vi "Read 2019 SweepControl JSON.vi"(8 "error in (no error)":errorcluster, 11 "json file":path) -> (0 "error out":errorcluster, 3 "data":T1)   [LabVIEW 2016]
uses:
  <vilib>/addons/_JKI.lib/Serialization/JSON/JKI JSON Serialization.lvlib
panel:
  out "text":string
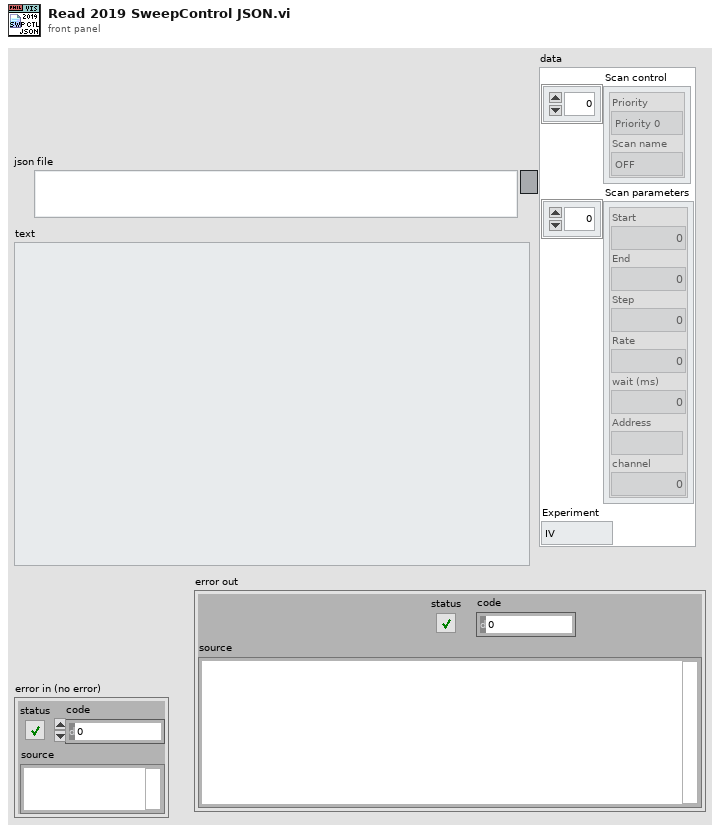
[diagram p1: front panel]
types:
  T1 = cluster{"Scan control":cluster{"Priority":enum16{"Priority 0", "Priority 1", "Priority 2", "Priority 3", "Priority 4", "Priority 5"}, "Scan name":enum16{"OFF", "DSA_Vsg2", "DSA_Vsg3", "DSA_Vbg", "DSA_Vsg1", "DSA_freq", "DSA_Vamp", "time", "Lockin Amplitude", "Lockin Frequency", "Lockin Bias", "Delay", "Strain", "DAQ Bias", "Magnet Field", "Temperature", "MW f1", "MW f2", "MW Amplitude1", "MW Amplitude2"}}[], "Scan parameters":cluster{"Start":dbl, "End":dbl, "Step":dbl, "Rate":dbl, "wait (ms)":u32, "Address":string, "channel":i32}[], "Experiment":enum16{"IV", "IV_Fast", "IV_Sweep", "THz_DelayLine", "Lockin_Vsg", "Lockin_Sweep", "Lockin_Time", "AI WFM time", "Lockin (experimental)"}}
  T2 = cluster{"Scan control":cluster{"Priority":enum16{"Priority 0", "Priority 1", "Priority 2", "Priority 3", "Priority 4", "Priority 5"}, "Scan name":enum16{"OFF", "DSA_Vsg2", "DSA_Vbg", "DSA_Vsg1", "DSA_freq", "DSA_Vamp", "time", "Lockin Amplitude", "Lockin Frequency", "Lockin Bias", "Delay", "Strain", "DAQ Bias", "Magnet Field", "Temperature", "MW f1", "MW f2", "MW Amplitude1", "MW Amplitude2"}}[], "Scan parameters":cluster{"Start":dbl, "End":dbl, "Step":dbl, "Rate":dbl, "wait (ms)":u32, "Address":string, "channel":i32}[], "Experiment":enum16{"IV", "IV_Fast", "IV_Sweep", "THz_DelayLine", "Lockin_Vsg", "Lockin_Sweep", "Lockin_Time", "AI WFM time", "Lockin (experimental)"}}
  T3 = cluster{"Experiment":enum16{"IV", "IV_Fast", "IV_Sweep", "THz_DelayLine", "Lockin_Vsg", "Lockin_Sweep", "Lockin_Time", "AI WFM time", "Lockin (experimental)"}, "Repeat Experiment":i32, "Scan control":cluster{"Priority":enum16{"Priority 0", "Priority 1", "Priority 2", "Priority 3", "Priority 4", "Priority 5"}, "Scan name":enum16{"OFF", "time", "Lockin Amplitude", "Lockin Frequency", "Lockin Bias", "Delay", "Strain", "DAQ Bias", "Magnet Field", "Temperature", "MW f1", "MW f2", "MW Amplitude1", "MW Amplitude2"}}[], "Scan parameters":cluster{"Start":dbl, "End":dbl, "Step":dbl, "Rate":dbl, "wait (ms/mK)":u32, "Address":string, "channel":i32}[]}
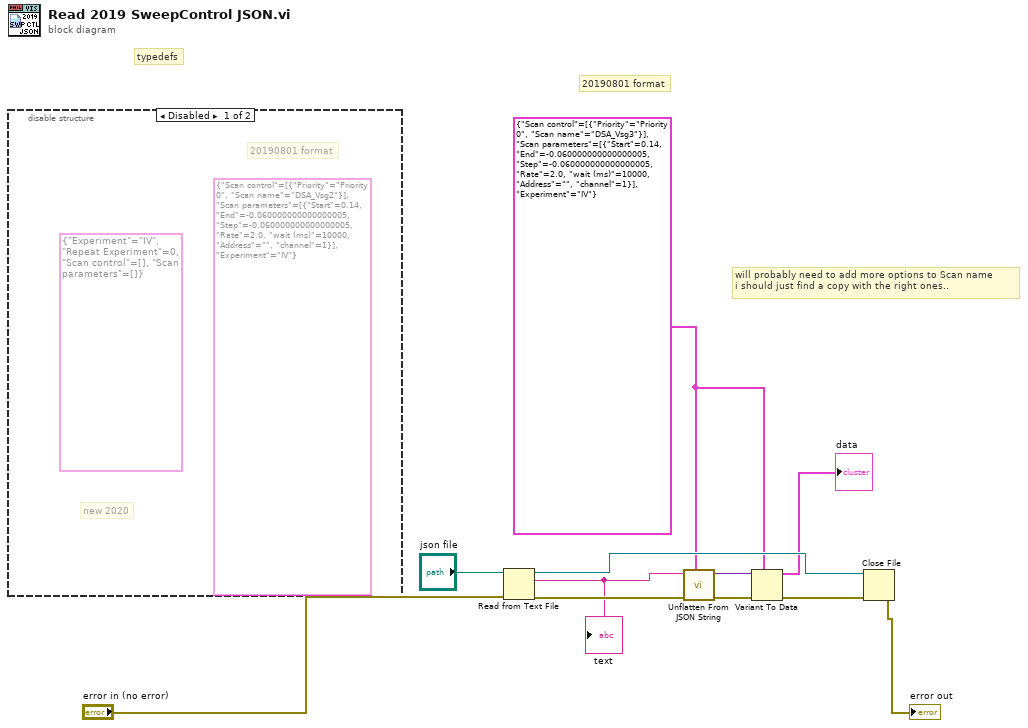
[diagram p0: block diagram]
diagram:
  w4 = T1 {"Scan control"=[{"Priority"=enum."Priority 0", "Scan name"=enum."DSA_Vsg3"}], "Scan parameters"=[{"Start"=0.14, "End"=-0.060000000000000005, "Step"=-0.060000000000000005, "Rate"=2.0, "wait (ms)"=10000, "Address"="", "channel"=1}], "Experiment"=enum."IV"} ("data")
  # "will probably need to add more options to Scan name\ni should just find a copy with the right ones.."
  # "20190801 format"
  # "typedefs"
  n1 = disable-structure shown="Disabled" {
    frame Disabled {
      (unwired) T2 {"Scan control"=[{"Priority"=enum."Priority 0", "Scan name"=enum."DSA_Vsg2"}], "Scan parameters"=[{"Start"=0.14, "End"=-0.060000000000000005, "Step"=-0.060000000000000005, "Rate"=2.0, "wait (ms)"=10000, "Address"="", "channel"=1}], "Experiment"=enum."IV"} ("data")
      (unwired) T3 {"Experiment"=enum."IV", "Repeat Experiment"=0, "Scan control"=[], "Scan parameters"=[]} ("data")
      # "20190801 format"
      # "new 2020"
    }
    frame Enabled {
    }
  }
  n2 = Read from Text File(file (use dialog)="json file", error in="error in (no error)") -> (refnum out=w7:refnum<file>, text=w6:string, error out=w11:errorcluster)  [unwired: 2 in, 1 out]
  "text" <- w6
  n3 = call <vilib>:"Unflatten From JSON String.vi"("Type and Defaults"=w4, "error in (no error)"=w11, "JSON String"=w6) -> ("error out"=w3:errorcluster, "Variant"=w5:variant)  [unwired: 7 in]
  n4 = Variant To Data(error in=w3, type=w4, Variant=w5) -> (data=→"data":T1, error out=w2:errorcluster)
  n5 = Close File(refnum=w7, error in=w2) -> (error out=→"error out":errorcluster)  [unwired: 1 out]
